vi "Pre-Build VI - Run Unit Tests.vi"(8 "error in (no error)":errorcluster) -> (0 "error out":errorcluster, 1 "VIs without test coverage":string[](array[string]), 2 "error type":enum16{"fatal", "non-fatal", "warning"}(ring), 3 "num tests":i32, 4 "VIs not loadable":string[](array[string]), 5 "VIs Failed":string[](array[string]))   [LabVIEW 2020]
uses:
  <vilib>/Utility/miscctls.llb/LVBookmarkInfoTypeDef.ctl
panel:
  out "VIs with #todo bookmarks":string[](array[string])
  out "VIs with #todo's":map{path, T1}(c390)
  out "VIs Succeeded":string[](array[string])
  in  "type specifier VI Refnum (for type only)":refnum<vi>
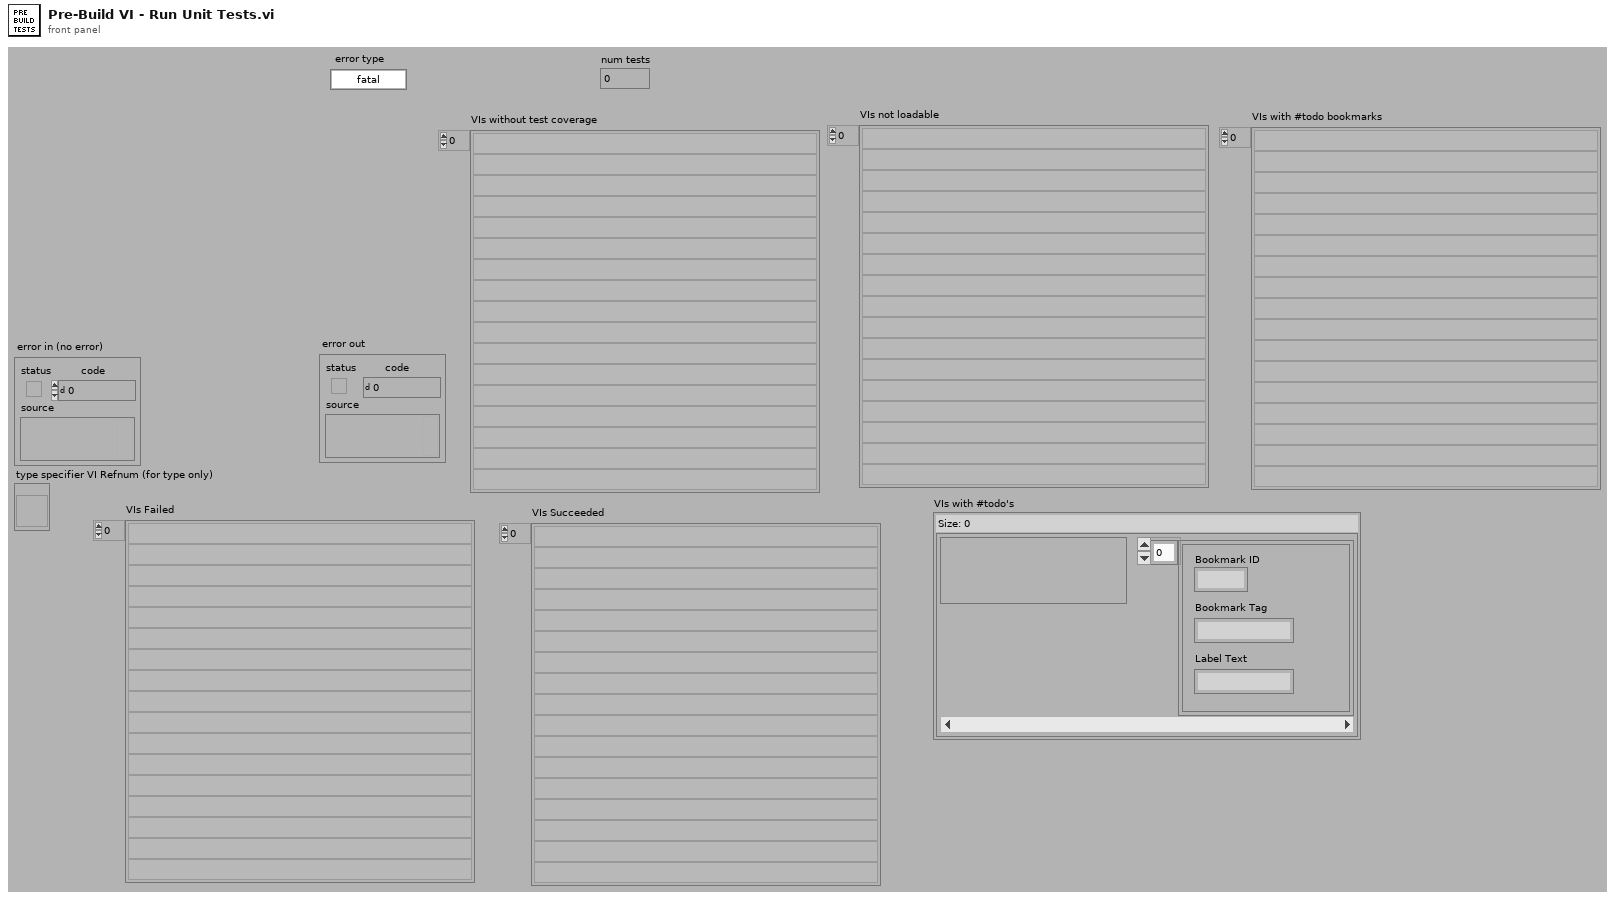
[diagram p1: front panel]
types:
  T1 = typedef "LVBookmarkInfoTypeDef.ctl" = cluster{"Bookmark ID":u32, "Bookmark Tag":string, "Label Text":string}[]
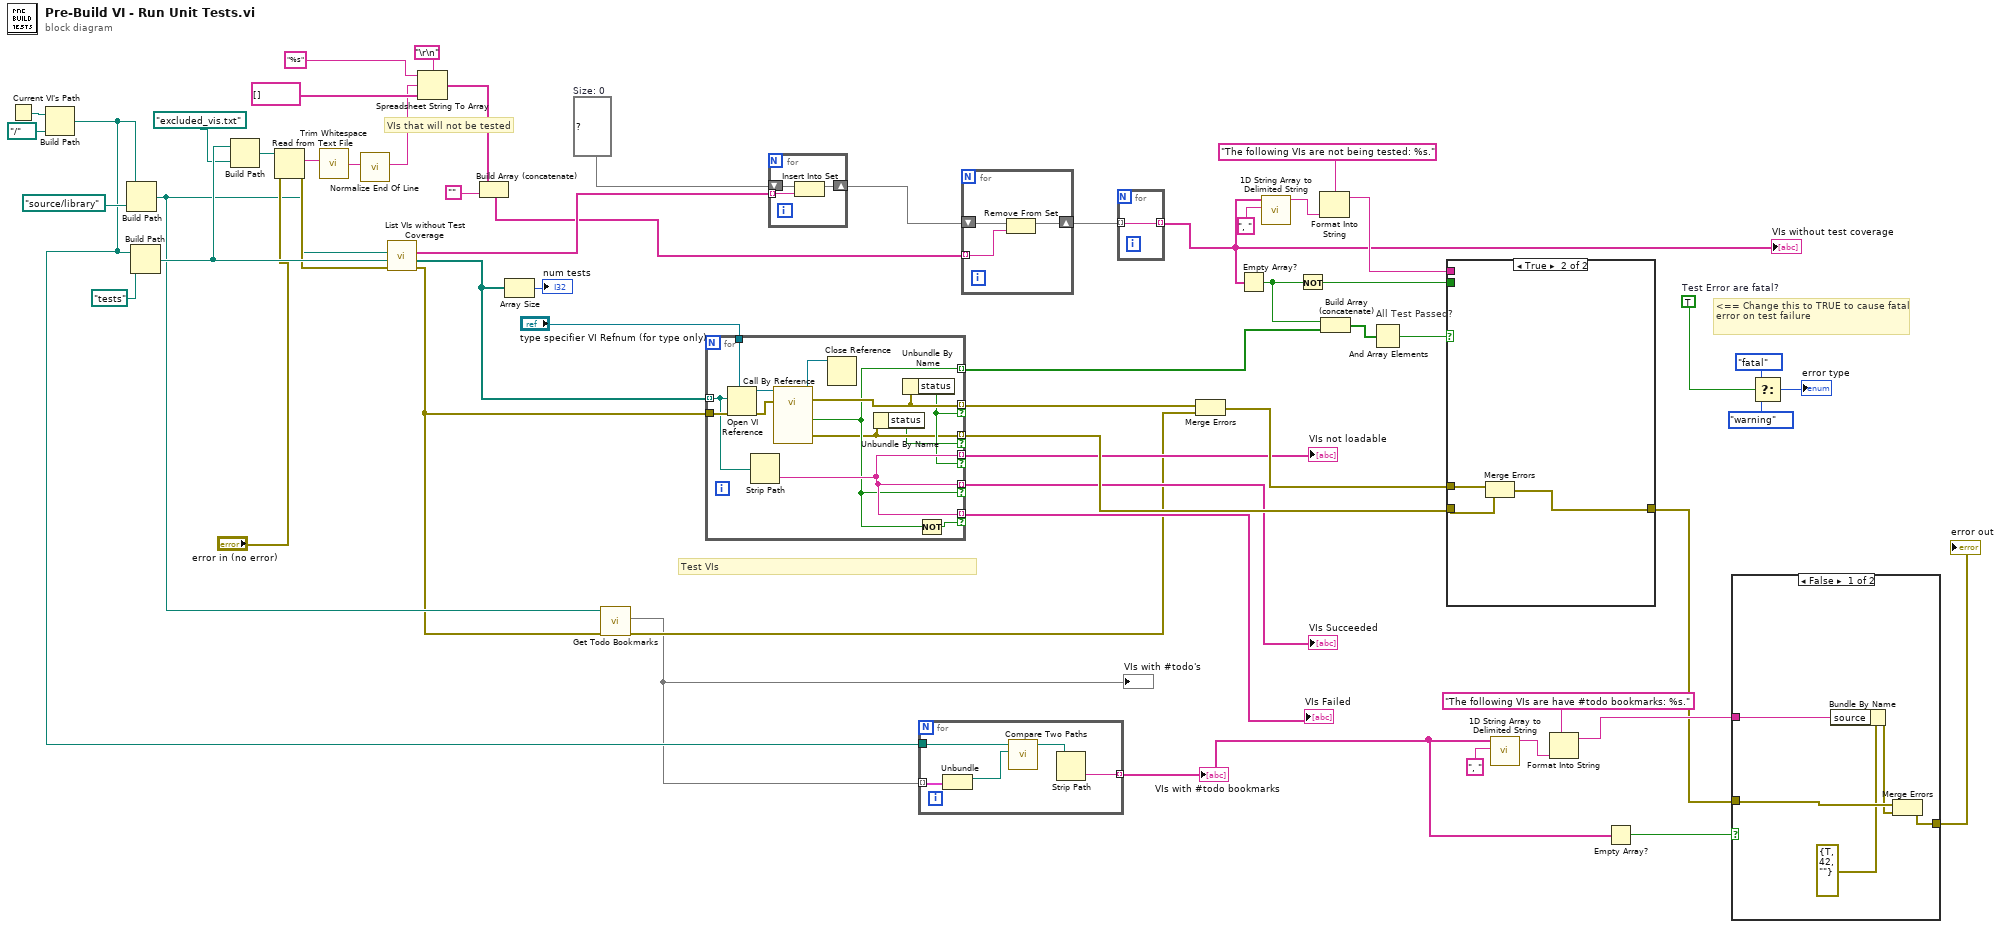
[diagram p0: block diagram]
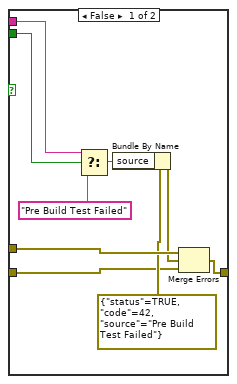
[diagram p3: hidden frame]
diagram:
  w31 = set{string} {}  # Size: 0
  w51 = TRUE  # Test Error are fatal?
  # "VIs that will not be tested"
  # "<== Change this to TRUE to cause fatal error on test failure"
  # "All Test Passed?"
  # "Test VIs"
  n1 = Current VI's Path() -> (path=w38:path)
  n2 = Build Path(base path=w38, name or relative path=path "../..") -> (appended path=w10:path)
  n3 = Build Path(base path=w10, name or relative path=path "source/library" ("Relative path (.)")) -> (appended path=w14:path)
  n4 = Build Path(base path=w10, name or relative path=path "tests" ("Relative path (.)")) -> (appended path=w34:path)
  n5 = Build Path(base path=w34, name or relative path=path "excluded_vis.txt" ("Relative path (.)")) -> (appended path=w32:path)
  n6 = Read from Text File(file (use dialog)=w32, error in="error in (no error)") -> (text=w19:string, error out=w17:errorcluster)  [unwired: 2 in, 2 out]
  n7 = call <vilib>:"Trim Whitespace.vi"("string"=w19) -> ("trimmed string"=w21:string)  [unwired: 1 in]
  n8 = call <vilib>:"Normalize End Of Line.vi"("string in"=w21) -> ("string out"=w20:string)  [unwired: 7 in]
  n9 = call "List VIs without Test Coverage.vi"("error in (no error)"=w17, "Tests Root"=w34, "Source Root"=w14) -> ("error out"=w11:errorcluster, "Test VIs"=w16:path[], "VIs without test coverage"=w30:string[])  [unwired: 6 in]
  n10 = Spreadsheet String To Array(delimiter (Tab)="\r\n", format string="%s", spreadsheet string=w20, array type (2D Dbl)=string[] [] ("appended array")) -> (array=w22:string[])
  n11 = Build Array (concatenate)(w22, "") -> (w28:string[])
  n12 = Array Size(array=w16) -> (size(s)=→"num tests":i32)
  n13 = call "Get Todo Bookmarks.vi"("error in (no error)"=w11, "Directory to Search"=w14) -> ("error out"=w13:errorcluster, "todo bookmarks"=w1:map{path, T1})  [unwired: 8 in]
  "VIs with #todo's" <- w1
  n14 = for {
    tunnel: w16 -> [w65] mode=indexing
    tunnel: "type specifier VI Refnum (for type only)" -> [w71]
    tunnel: [w63] -> w42 mode=indexing
    tunnel: [w60] -> w46 mode=indexing if=w59
    tunnel: w11 -> [w67]
    tunnel: [w66] -> w43 mode=indexing if=w61
    tunnel: [w64] -> w41 mode=indexing if=w61
    tunnel: [w64] -> w40 mode=indexing if=w63
    tunnel: [w64] -> w39 mode=indexing if=w62
    n15 = Open VI Reference(type specifier VI Refnum (for type only)=w71, vi path=w65, error in (no error)=w67) -> (vi reference=w70:refnum<vi>, error out=w69:errorcluster)  [unwired: 3 in]
    n16 = Strip Path(path=w65) -> (name=w64:string)  [unwired: 1 out]
    n17 = call-by-ref "?"(reference=w70, error in=w69) -> (reference out=w68:refnum<vi>, error out=w66:errorcluster, 0:"error out"=w60:errorcluster, "pass"=w63:bool)  [unwired: 10 in]
    n18 = Close Reference(reference=w68) -> ()  [unwired: 1 in, 1 out]
    n19 = Unbundle By Name(w60) -> ("status"=w59:bool)
    n20 = Unbundle By Name(w66) -> ("status"=w61:bool)
    n21 = Not(x=w63) -> (.not. x?=w62:bool)
  }
  "VIs not loadable" <- w41
  "VIs Succeeded" <- w40
  "VIs Failed" <- w39
  n22 = for {
    tunnel: w30 -> [w74] mode=indexing
    shift-right: [w72] -> w29
    shift-left: w31 -> [w73]
    n23 = Insert Into Set(10:w74, 11:w73) -> (3:w72:set{string})  [unwired: 1 out]
  }
  n24 = for {
    tunnel: w1 -> [w79] mode=indexing
    tunnel: w10 -> [w77]
    tunnel: [w75] -> w5 mode=indexing
    n25 = Unbundle(w79) -> ("key type"=w78:path)  [unwired: 1 out]
    n26 = call <vilib>:"Compare Two Paths.vi"("Path 2"=w78, "Path 1"=w77) -> ("Relative Path from 1 to 2"=w76:path)  [unwired: 6 in, 3 out]
    n27 = Strip Path(path=w76) -> (name=w75:string)  [unwired: 1 out]
  }
  "VIs with #todo bookmarks" <- w5
  n28 = for {
    shift-right: [w80] -> w27
    shift-left: w29 -> [w82]
    tunnel: w28 -> [w81] mode=indexing
    n29 = Remove From Set(10:w81, 11:w82) -> (3:w80:set{string})  [unwired: 1 out]
  }
  n30 = for {
    tunnel: [w83] -> w26 mode=indexing
    tunnel: w27 -> [w83] mode=indexing
  }
  "VIs without test coverage" <- w26
  n31 = Merge Errors(w43, w13) -> (w44:errorcluster)
  n32 = Empty Array?(array=w26) -> (empty?=w53:bool)
  n33 = call <vilib>:"1D String Array to Delimited String.vi"("delimiter"=", " ("delimiter (Tab)"), "string array"=w26) -> ("delimited string"=w56:string)  [unwired: 9 in]
  n34 = Not(x=w53) -> (.not. x?=w52:bool)
  n35 = Format Into String(format string="The following VIs are not being tested: %s.", w56) -> (resulting string=w54:string)  [unwired: 2 in, 1 out]
  n36 = Build Array (concatenate)(w53, w42) -> (w12:bool[])
  n37 = And Array Elements(Boolean array=w12) -> (logical AND=w58:bool)
  n38 = case shown="True" w58 {
    tunnel: w44 -> [w92 w95]
    tunnel: [w91 w94] -> w2
    tunnel: w52 -> [w90 _]
    tunnel: w54 -> [w89 _]
    tunnel: w46 -> [w84 w93]
    frame False {
      n39 = Select(t=w89, s=w90, f="Pre Build Test Failed" ("source")) -> (s? t:f=w87:string)
      n40 = Bundle By Name(cluster=errorcluster {"status"=TRUE, "code"=42, "source"="Pre Build Test Failed"} ("error out"), "source"=w87) -> (w86:errorcluster)
      n41 = Merge Errors(w92, w86, w84) -> (w91:errorcluster)
    }
    frame True {
      n42 = Merge Errors(w95, w93) -> (w94:errorcluster)
    }
  }
  n43 = call <vilib>:"1D String Array to Delimited String.vi"("delimiter"=", " ("delimiter (Tab)"), "string array"=w5) -> ("delimited string"=w8:string)  [unwired: 9 in]
  n44 = Format Into String(format string="The following VIs are have #todo bookmarks: %s.", w8) -> (resulting string=w6:string)  [unwired: 2 in, 1 out]
  n45 = Empty Array?(array=w5) -> (empty?=w4:bool)
  n46 = case shown="False" w4 {
    tunnel: w2 -> [w100 w101]
    tunnel: [w96 w101] -> w3
    tunnel: w6 -> [w97 _]
    frame False {
      n47 = Bundle By Name(cluster=errorcluster {"status"=TRUE, "code"=42, "source"=""} ("error out"), "source"=w97) -> (w99:errorcluster)
      n48 = Merge Errors(w100, w99) -> (w96:errorcluster)
    }
    frame True {
    }
  }
  "error out" <- w3
  n49 = Select(t=enum16{"fatal", "non-fatal", "warning"}."fatal" ("error type"), s=w51, f=enum16{"fatal", "non-fatal", "warning"}."warning" ("error type")) -> (s? t:f=→"error type":enum16{"fatal", "non-fatal", "warning"})
